vi "Test Bench.vi"() -> ()   [LabVIEW 2018]
uses:
  RT Parameters/RT Parameter.ctl
  RT Parameters/RT Experiments.ctl
  RT Parameters/RT Mass Range.ctl
  RT Parameters/RT Active Ch.ctl
  RT Parameters/RT Res Type.ctl
  RT Parameters/RT Run Mode.ctl
panel:
  in  "RT Parameter":T1 {"Expt"."Mass Range"."Resolution Type" items=["High/High", "Medium/Medium", "Low/Low", "High/Medium", "High/Low", "Medium/High", "Medium/Low", "Low/High", "Low/Medium"]}
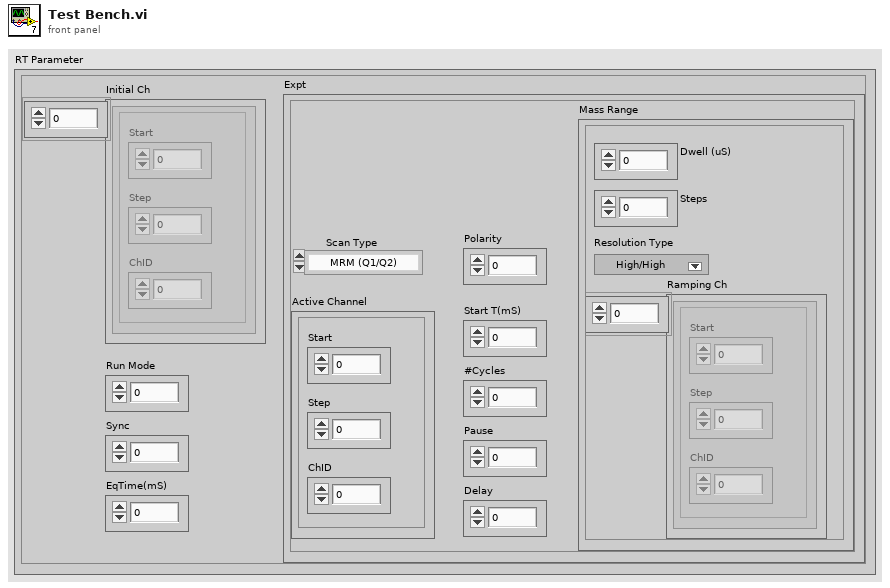
[diagram p1: front panel]
types:
  T1 = typedef "RT Parameter.ctl" = cluster{"Expt":T2, "Initial Ch":T4[], "Run Mode":i32, "Sync":u8, "EqTime(mS)":i32}
  T2 = typedef "RT Experiments.ctl" = cluster{"Mass Range":T3, "Active Channel":T4, "Scan Type":T6, "Polarity":u8, "Start T(mS)":i32, "#Cycles":i32, "Pause":i32, "Delay":i32}
  T3 = typedef "RT Mass Range.ctl" = cluster{"Ramping Ch":T4[], "Resolution Type":T5, "Steps":dbl, "Dwell (uS)":dbl}
  T4 = typedef "RT Active Ch.ctl" = cluster{"Start":dbl, "Step":dbl, "ChID":dbl}
  T5 = typedef "RT Res Type.ctl" = u16
  T6 = typedef "RT Run Mode.ctl" = enum16{"MRM (Q1/Q2)", "Q1 Scan", "Q1 SRM", "Q2 Scan", "Q2 SRM", "Product Scan", "Precursor Scan", "Neutral Loss", "Neutral Gain"}
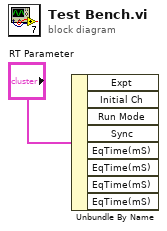
[diagram p0: block diagram]
diagram:
  n1 = Unbundle By Name("RT Parameter") -> ()  [unwired: 8 out]
